vi "MPPT Silicon model.vi"() -> ()   [LabVIEW 2020]
doc: "This example shows how to create, run a script and query the script output data."
panel:
  out "Start Time":string
  out "Time(Min)":dbl[](array[numeric]) format="%#_8g"
  out "P Vs T":cluster{dbl[], dbl[]}(graph)
  out "Iteration No.":i32
  in  "Delay(s)":u32=5
  out "Current":dbl[](array[numeric])
  out "P, I Vs V":cluster{dbl[], dbl[]}[](graph)
  out "P(k-1)":dbl
  out "P(k)":dbl
  out "V(k-1)":dbl
  out "V(k)":dbl
  out "Voltage":dbl[](array[numeric])
  out "Power":dbl[](array[numeric])
  in  "stop":bool
  in  "dV":dbl=0.1 caption="limitI"
  in  "Initial Voltage (V)":dbl caption="limitI"
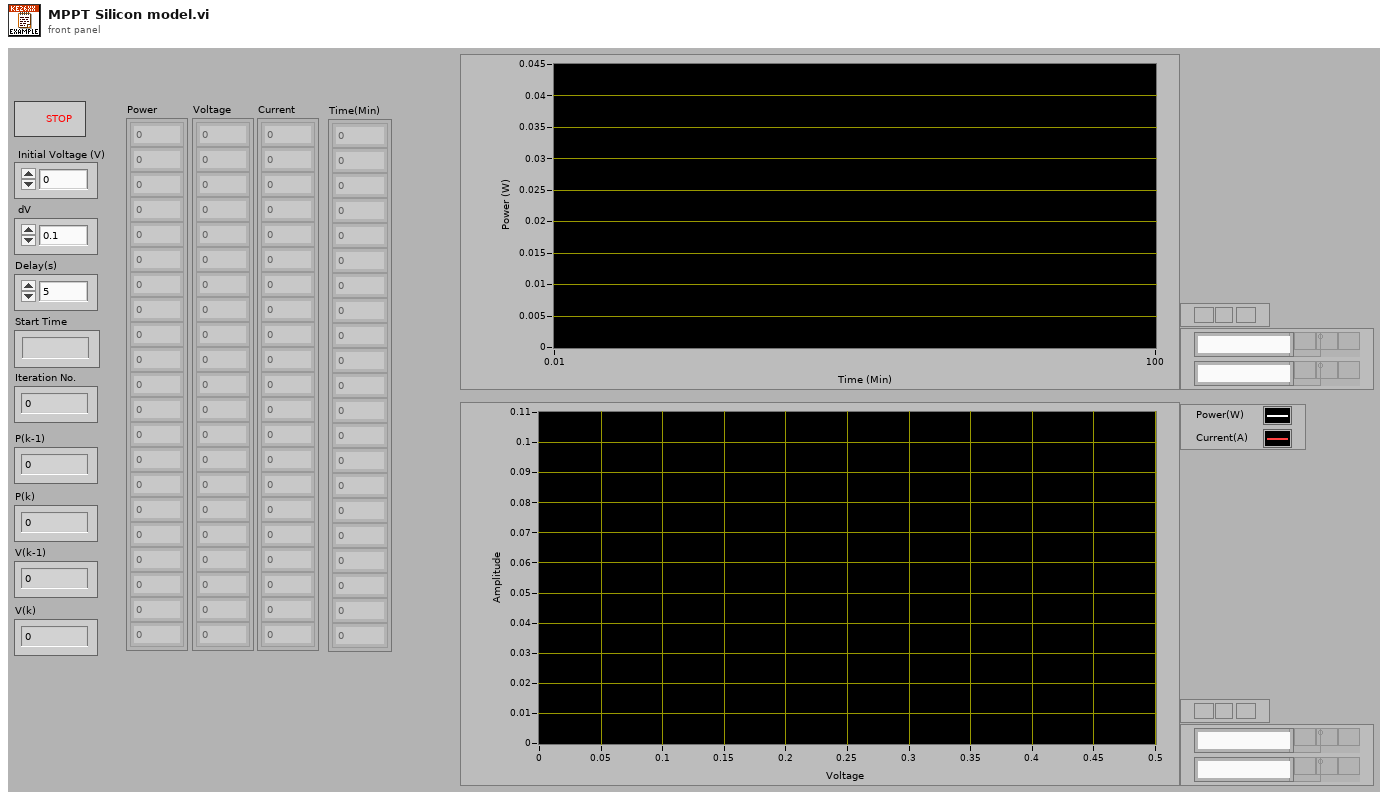
[diagram p1: front panel]
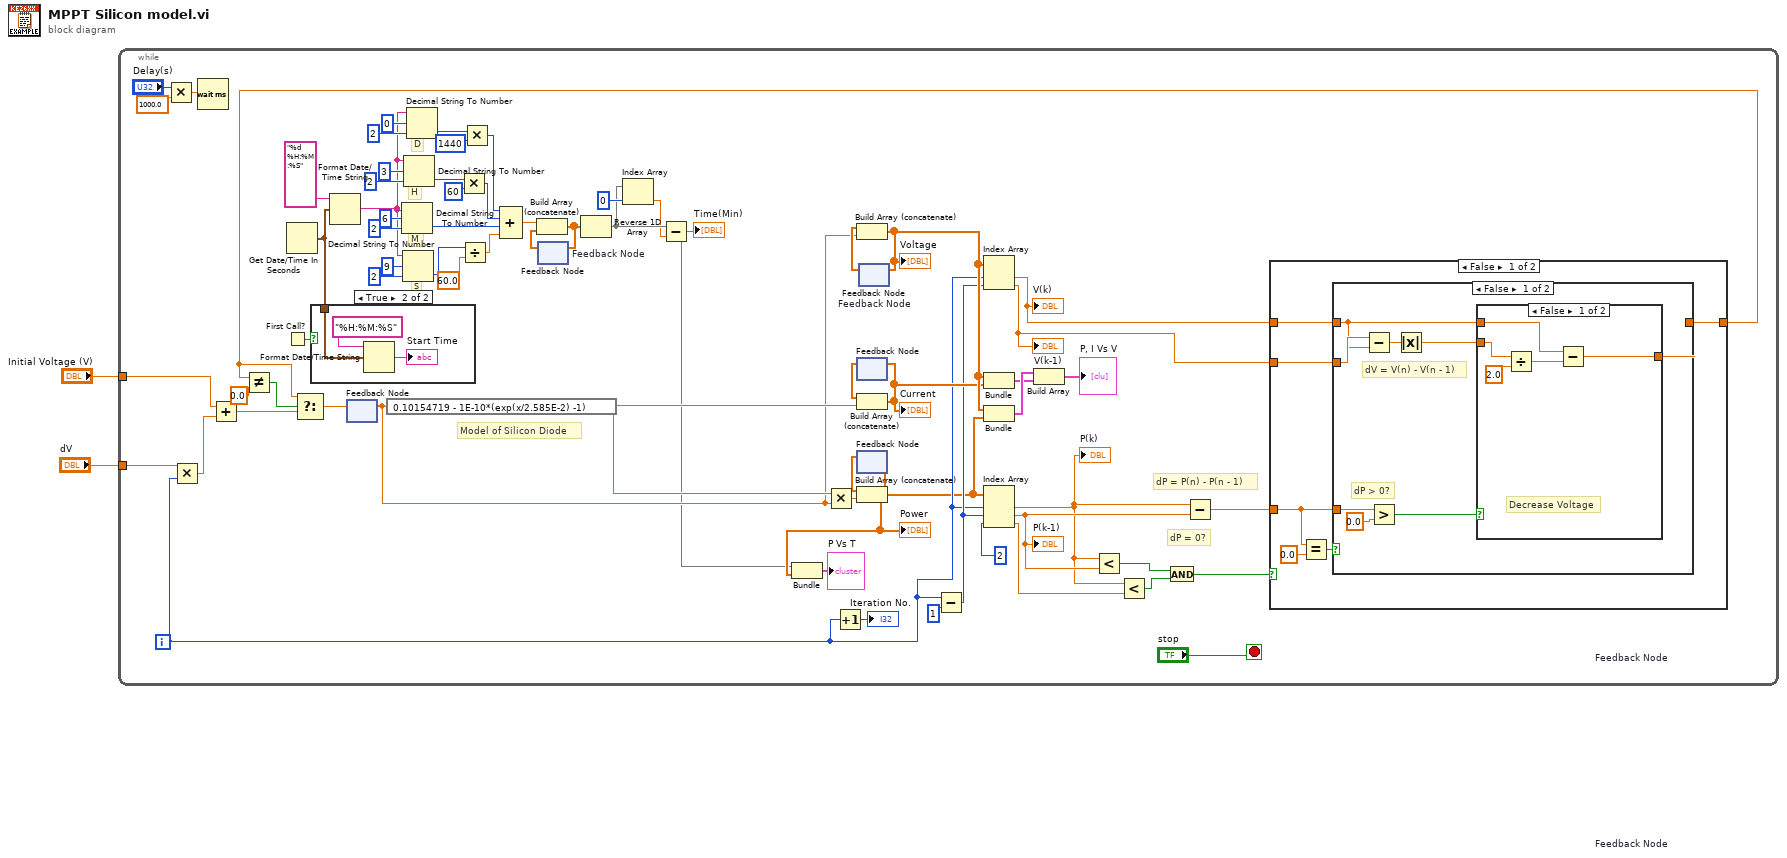
[diagram p0: block diagram]
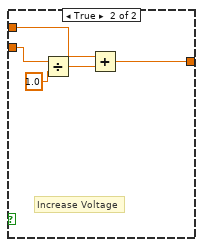
[diagram p3: hidden frame]
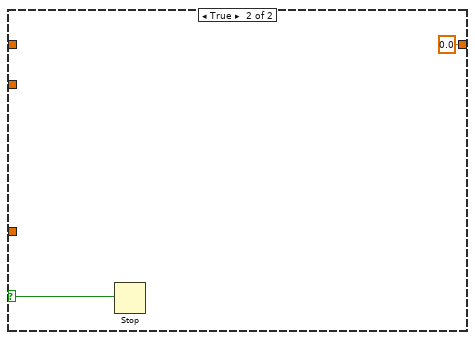
[diagram p5: hidden frame]
diagram:
  n1 = while {
    tunnel: "dV" -> [w70]
    tunnel: "Initial Voltage (V)" -> [w68]
    i -> [w39]
    stop <- "stop" stop-if-true
    # "D"
    # "H"
    # "M"
    # "S"
    # "dP = 0?"
    # "dP = P(n) - P(n - 1)"
    # "Model of Silicon Diode"
    n2 = Multiply(x="Delay(s)", y=1000.0) -> (x*y=w4:dbl)
    n3 = Multiply(x=w70, y=w39) -> (x*y=w69:dbl)
    n4 = Wait (ms)(milliseconds to wait=w4) -> ()  [unwired: 1 out]
    n5 = Add(x=w68, y=w69) -> (x+y=w44:dbl)
    n6 = First Call?() -> (First Call?: T/F=w8:bool)
    n7 = Get Date/Time In Seconds() -> (seconds since 1Jan1904=w9:timestamp)
    n8 = case shown="True" w8 {
      tunnel: w9 -> [_ w72]
      frame False {
      }
      frame True {
        n9 = Format Date/Time String(time format string (%c)="%H:%M:%S", seconds (now)=w72) -> (date/time string=→"Start Time":string)  [unwired: 1 out]
      }
    }
    n10 = Format Date/Time String(time format string (%c)="%d %H:%M:%S", seconds (now)=w9) -> (date/time string=w18:string)  [unwired: 1 out]
    n11 = feedback #1() -> (w29:dbl)  [unwired: 1 in]
    n12 = expression code="0.10154719 - 1E-10*(exp(x/2.585E-2) -1)"(w29) -> (w64:dbl)
    n13 = Decimal String To Number(string=w18, offset=6 ("offset (0)"), default (0L)=2 ("length (rest)")) -> (number=w28:i32)  [unwired: 1 out]
    n14 = Decimal String To Number(string=w18, offset=9 ("offset (0)"), default (0L)=2 ("length (rest)")) -> (number=w27:i32)  [unwired: 1 out]
    n15 = Decimal String To Number(string=w18, offset=3 ("offset (0)"), default (0L)=2 ("length (rest)")) -> (number=w24:i32)  [unwired: 1 out]
    n16 = Decimal String To Number(string=w18, offset=0 ("offset (0)"), default (0L)=2 ("length (rest)")) -> (number=w21:i32)  [unwired: 1 out]
    n17 = Multiply(x=w24, y=60) -> (x*y=w25:i32)
    n18 = Divide(x=w27, y=60.0) -> (x/y=w26:dbl)
    n19 = Multiply(x=w21, y=1440) -> (x*y=w17:i32)
    n20 = Compound Arithmetic op=ADD(w17, w25, w28, w26) -> (w14:dbl)
    n21 = feedback #2 "Feedback Node"() -> (w15:dbl[])  [unwired: 1 in]
    n22 = Build Array (concatenate)(w14, w15) -> (w13:dbl[])
    n23 = feedback-in #2(w13) -> ()
    n24 = Reverse 1D Array(array=w13) -> (reversed array=w11:dbl[])
    n25 = Index Array(array=w11, index=0) -> (element=w10:dbl)
    n26 = Subtract(x=w11, y=w10) -> (x-y=w7:dbl[])
    "Time(Min)" <- w7
    n27 = Multiply(x=w64, y=w29) -> (x*y=w66:dbl)
    n28 = Increment(x=w39) -> (x+1=→"Iteration No.":i32)
    n29 = feedback #3 "Feedback Node"() -> (w65:dbl[])  [unwired: 1 in]
    n30 = Build Array (concatenate)(w65, w64) -> (w58:dbl[])
    "Current" <- w58
    n31 = feedback-in #3(w58) -> ()
    n32 = feedback #4 "Feedback Node"() -> (w67:dbl[])  [unwired: 1 in]
    n33 = Build Array (concatenate)(w67, w66) -> (w37:dbl[])
    "Power" <- w37
    n34 = Bundle(w7, w37) -> (→"P Vs T":cluster{dbl[], dbl[]})  [unwired: 1 in]
    n35 = feedback-in #4(w37) -> ()
    n36 = feedback #5 "Feedback Node"() -> (w63:dbl[])  [unwired: 1 in]
    n37 = Build Array (concatenate)(w63, w29) -> (w62:dbl[])
    "Voltage" <- w62
    n38 = feedback-in #5(w62) -> ()
    n39 = Subtract(x=w39, y=1) -> (x-y=w56:i32)
    n40 = Index Array(array=w62, index #1=w39, index #2=w56) -> (element #1=w55:dbl, element #2=w40:dbl)
    "V(k)" <- w55
    "V(k-1)" <- w40
    n41 = Bundle(w62, w58) -> (w60:cluster{dbl[], dbl[]})  [unwired: 1 in]
    n42 = Bundle(w62, w37) -> (w61:cluster{dbl[], dbl[]})  [unwired: 1 in]
    n43 = Index Array(array=w37, index #1=w39, index #2=w56, index #3=2 ("index")) -> (element #1=w49:dbl, element #2=w53:dbl, element #3=w48:dbl)
    "P(k)" <- w49
    "P(k-1)" <- w53
    n44 = Build Array(w61, w60) -> (→"P, I Vs V":cluster{dbl[], dbl[]}[])
    n45 = Less?(x=w49, y=w53) -> (x < y?=w51:bool)
    n46 = Less?(x=w49, y=w48) -> (x < y?=w50:bool)
    n47 = And(x=w51, y=w50) -> (x .and. y?=w52:bool)
    n48 = Subtract(x=w49, y=w53) -> (x-y=w54:dbl)
    n49 = case shown="False" w52 {
      selector: w52 -> [_ w99]
      tunnel: w55 -> [w79 _]
      tunnel: w40 -> [w78 _]
      tunnel: w54 -> [w75 _]
      tunnel: [w77 0.0] -> w42
      frame False {
        n50 = Equal?(x=w75, y=0.0) -> (x = y?=w74:bool)
        n51 = case shown="False" w74 {
          tunnel: w79 -> [w80 w98]
          tunnel: w78 -> [w83 _]
          tunnel: [w84 w98] -> w77
          tunnel: w75 -> [w85 _]
          frame False {
            # "dV = V(n) - V(n - 1)"
            # "dP > 0?"
            n52 = Subtract(x=w83, y=w80) -> (x-y=w82:dbl)
            n53 = Greater?(x=w85, y=0.0) -> (0:w86:bool)
            n54 = Absolute Value(x=w82) -> (abs(x)=w81:dbl)
            n55 = case shown="False" w86 {
              tunnel: [w90 w95] -> w84
              tunnel: w81 -> [w92 w96]
              tunnel: w80 -> [w91 w97]
              frame False {
                # "Decrease Voltage"
                n56 = Divide(x=w92, y=2.0) -> (x/y=w89:dbl)
                n57 = Subtract(x=w91, y=w89) -> (x-y=w90:dbl)
              }
              frame True {
                # "Increase Voltage"
                n58 = Divide(x=w96, y=1.0) -> (x/y=w94:dbl)
                n59 = Add(x=w97, y=w94) -> (x+y=w95:dbl)
              }
            }
          }
          frame True {
          }
        }
      }
      frame True {
        n60 = Stop(stop? (T)=w99) -> ()
      }
    }
    n61 = Not Equal?(x=w42, y=0.0) -> (x != y?=w43:bool)
    n62 = Select(t=w42, s=w43, f=w44) -> (s? t:f=w41:dbl)
    n63 = feedback-in #1(w41) -> ()
  }
